vi "Next floor logic.vi"(9 "Elevator states array":T1[](array[typedef]), 11 "Floors to serve":i32[](array[numeric])) -> (1 "Elevator states array out":T1[](array[typedef]), 3 "Floors to serve out":i32[](array[numeric]))   [LabVIEW 2019]
uses:
  Type defs/Elevator states.ctl
  Type defs/Elevator position.ctl
  Type defs/Car buttons.ctl
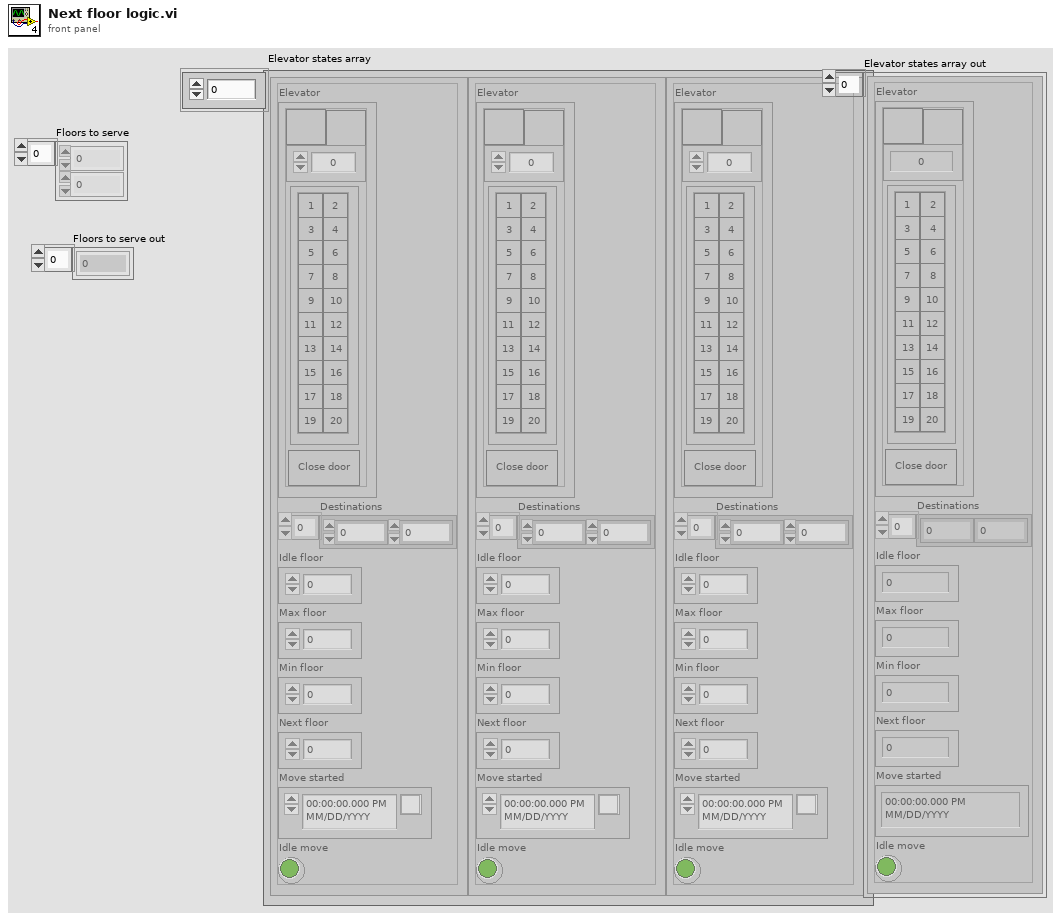
[diagram p1: front panel]
types:
  T1 = typedef "Elevator states.ctl" = cluster{"Elevator":T2, "Destinations":i32[], "Idle floor":u16, "Max floor":u16, "Min floor":u16, "Next floor":u16, "Move started":timestamp, "Idle move":bool}
  T2 = typedef "Elevator position.ctl" = cluster{"Up Button":bool, "Current floor":u16, "Down Button":bool, "Car":T3, "Close door":bool}
  T3 = typedef "Car buttons.ctl" = cluster{"Blank Button":bool, "Blank Button 2":bool, "Blank Button 3":bool, "Blank Button 4":bool, "Blank Button 5":bool, "Blank Button 6":bool, "Blank Button 7":bool, "Blank Button 8":bool, "Blank Button 9":bool, "Blank Button 10":bool, "Blank Button 11":bool, "Blank Button 12":bool, "Blank Button 13":bool, "Blank Button 14":bool, "Blank Button 15":bool, "Blank Button 16":bool, "Blank Button 17":bool, "Blank Button 18":bool, "Blank Button 19":bool, "Blank Button 20":bool}
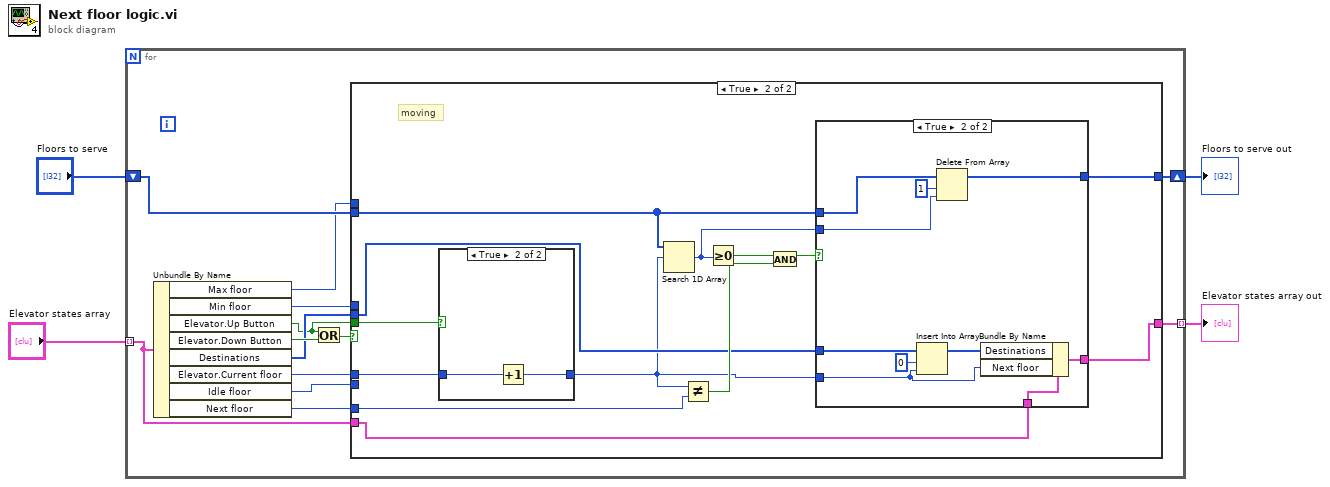
[diagram p0: block diagram]
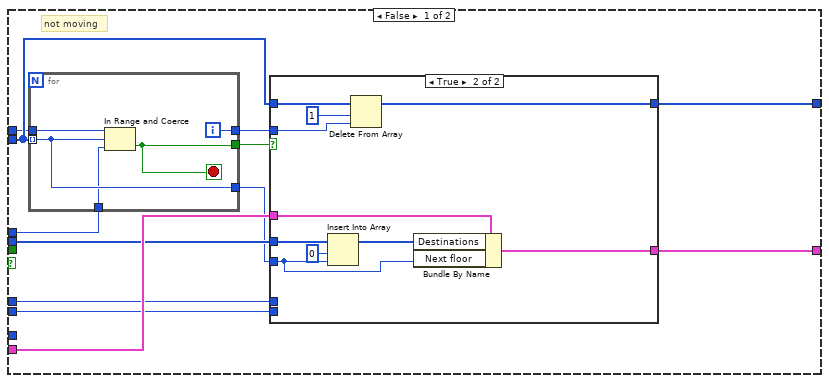
[diagram p2: hidden frame]
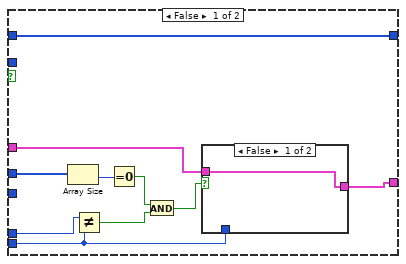
[diagram p3: hidden frame]
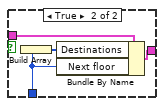
[diagram p4: hidden frame]
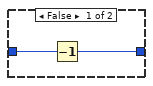
[diagram p6: hidden frame]
diagram:
  n1 = for {
    tunnel: "Elevator states array" -> [w14] mode=indexing
    shift-right: [w12] -> w2
    shift-left: "Floors to serve" -> [w15]
    tunnel: [w11] -> w1 mode=indexing
    n2 = Unbundle By Name(w14) -> ("Max floor"=w10:u16, "Min floor"=w9:u16, "Elevator.Up Button"=w6:bool, "Elevator.Down Button"=w17:bool, "Destinations"=w13:i32[], "Elevator.Current floor"=w8:u16, "Idle floor"=w7:u16, "Next floor"=w5:u16)
    n3 = Or(x=w6, y=w17) -> (x .or. y?=w16:bool)
    n4 = case shown="True" w16 {
      tunnel: w15 -> [w24 w64]
      tunnel: w14 -> [w28 w69]
      tunnel: w13 -> [w27 w65]
      tunnel: [w22 w62] -> w12
      tunnel: [w25 w60] -> w11
      tunnel: w10 -> [w21 _]
      tunnel: w9 -> [w20 _]
      tunnel: w8 -> [w19 w71]
      tunnel: w7 -> [w18 _]
      tunnel: w6 -> [_ w72]
      tunnel: w5 -> [_ w68]
      frame False {
        # "not moving"
        n5 = for {
          tunnel: w24 -> [w58] mode=indexing
          tunnel: [w59] -> w29
          tunnel: [w58] -> w26
          tunnel: [w57] -> w23
          tunnel: w21 -> [w56]
          tunnel: w20 -> [w55]
          i -> [w57]
          stop <- w59 stop-if-true
          n6 = In Range and Coerce(upper limit=w56, x=w58, lower limit=w55) -> (In Range?=w59:bool)  [unwired: 1 out]
        }
        n7 = case shown="True" w29 {
          tunnel: w28 -> [w32 w54]
          tunnel: w27 -> [w38 w53]
          tunnel: w26 -> [_ w46]
          tunnel: [w31 w51] -> w25
          tunnel: w24 -> [w39 w49]
          tunnel: w23 -> [_ w48]
          tunnel: [w39 w47] -> w22
          tunnel: w19 -> [w36 _]
          tunnel: w18 -> [w30 _]
          frame False {
            n8 = Array Size(array=w38) -> (size(s)=w37:i32)
            n9 = Not Equal?(x=w36, y=w30) -> (x != y?=w34:bool)
            n10 = Equal To 0?(x=w37) -> (x = 0?=w35:bool)
            n11 = And(x=w35, y=w34) -> (x .and. y?=w33:bool)
            n12 = case shown="False" w33 {
              tunnel: w32 -> [w40 w44]
              tunnel: [w40 w43] -> w31
              tunnel: w30 -> [_ w41]
              frame False {
              }
              frame True {
                n13 = Build Array(w41) -> (w42:u16[])
                n14 = Bundle By Name(cluster=w44, "Destinations"=w42, "Next floor"=w41) -> (w43:T1)
              }
            }
          }
          frame True {
            n15 = Insert Into Array(array=w53, index=0, new element=w46) -> (w52:i32[])
            n16 = Delete From Array(array=w49, length=1, index=w48) -> (array with subset deleted=w47:i32[])  [unwired: 1 out]
            n17 = Bundle By Name(cluster=w54, "Destinations"=w52, "Next floor"=w46) -> (w51:T1)
          }
        }
      }
      frame True {
        # "moving"
        n18 = case shown="True" w72 {
          tunnel: w71 -> [w86 w88]
          tunnel: [w85 w87] -> w61
          frame False {
            n19 = Decrement(x=w86) -> (x-1=w85:u16)
          }
          frame True {
            n20 = Increment(x=w88) -> (x+1=w87:u16)
          }
        }
        n21 = Search 1D Array(1D array=w64, element=w61) -> (index of element=w63:i32)  [unwired: 1 in]
        n22 = Not Equal?(x=w61, y=w68) -> (x != y?=w66:bool)
        n23 = Greater Or Equal To 0?(x=w63) -> (x >= 0?=w70:bool)
        n24 = And(x=w70, y=w66) -> (x .and. y?=w67:bool)
        n25 = case shown="True" w67 {
          tunnel: w69 -> [w74 w84]
          tunnel: w65 -> [_ w83]
          tunnel: w64 -> [w73 w80]
          tunnel: w63 -> [_ w79]
          tunnel: [w73 w77] -> w62
          tunnel: w61 -> [_ w76]
          tunnel: [w74 w75] -> w60
          frame False {
          }
          frame True {
            n26 = Insert Into Array(array=w83, index=0, new element=w76) -> (w81:i32[])
            n27 = Delete From Array(array=w80, length=1, index=w79) -> (array with subset deleted=w77:i32[])  [unwired: 1 out]
            n28 = Bundle By Name(cluster=w84, "Destinations"=w81, "Next floor"=w76) -> (w75:T1)
          }
        }
      }
    }
  }
  "Floors to serve out" <- w2
  "Elevator states array out" <- w1
